vi "User New.vi"(1 "Existing User Records (empty)":T1[](array[typedef])) -> (0 "Default New User":T1)   [LabVIEW 2011]
uses:
  User Record.ctl
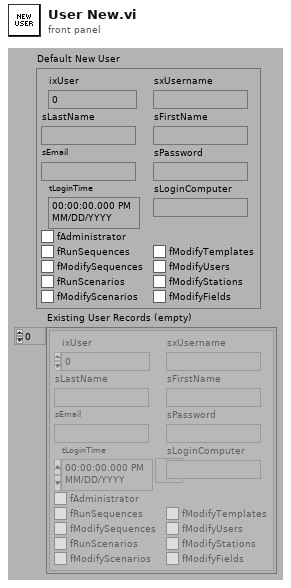
[diagram p1: front panel]
types:
  T1 = typedef "User Record.ctl" = cluster{"ixUser":i32, "sxUsername":string, "sLastName":string, "sFirstName":string, "sEmail":string, "sPassword":string, "tLoginTime":timestamp, "sLoginComputer":string, "fAdministrator":bool, "fRunSequences":bool, "fModifySequences":bool, "fRunScenarios":bool, "fModifyScenarios":bool, "fModifyTemplates":bool, "fModifyUsers":bool, "fModifyStations":bool, "fModifyFields":bool}
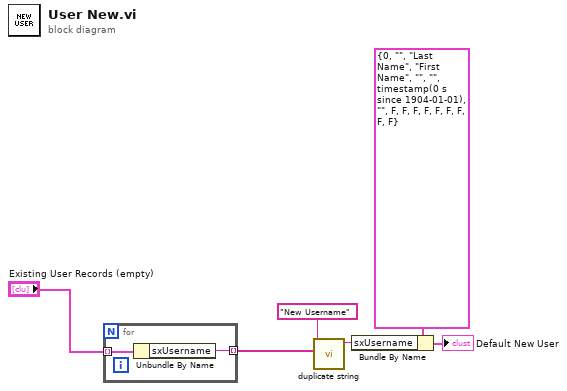
[diagram p0: block diagram]
diagram:
  n1 = for {
    tunnel: "Existing User Records (empty)" -> [w8] mode=indexing
    tunnel: [w7] -> w5 mode=indexing
    n2 = Unbundle By Name(w8) -> ("sxUsername"=w7:string)
  }
  n3 = call "duplicate string.vi"("Array of Strings"=w5, "String"="New Username") -> ("Updated String"=w2:string)  [unwired: 9 out]
  n4 = Bundle By Name(cluster=T1 {"ixUser"=0, "sxUsername"="", "sLastName"="Last Name", "sFirstName"="First Name", "sEmail"="", "sPassword"="", "tLoginTime"=timestamp(0 s since 1904-01-01), "sLoginComputer"="", "fAdministrator"=FALSE, "fRunSequences"=FALSE, "fModifySequences"=FALSE, "fRunScenarios"=FALSE, "fModifyScenarios"=FALSE, "fModifyTemplates"=FALSE, "fModifyUsers"=FALSE, "fModifyStations"=FALSE, "fModifyFields"=FALSE} ("Default New User"), "sxUsername"=w2) -> (→"Default New User":T1)
